vi "SMO.BasicByRef.GetValue.vi"(8 "error in (no error)":errorcluster, 11 "SMO.BasicByRef":refnum<class "SMO.BasicByRef.lvclass">) -> (0 "error out":errorcluster, 2 "Value":T1, 3 "SMO.BasicByRef out":refnum<class "SMO.BasicByRef.lvclass">)   [LabVIEW 2019, in "SMO.BasicByRef.lvclass"]
doc: "---------------------------------------------------------------\nJKI State Machine Objects™\nhttp://jki.net/state-machine-objects/\nCopyright (C) 2005-2015, JKI <info@jki.net>\nALL RIGHTS RESERVEDJKI State Machine Objects (SMO) 1.0.0.5\nJKI - JKI\nCopyright (c) 2016, JKI"
uses:
  SMO.BasicByRef.lvclass
  Typedefs/Value.ctl
  SMO.BasicByRef.lvclass/SMO.BasicByRef.ctl
panel:
  # "For instructions on how to use the JKI State Machine Objects, examples and video tutorials, visit:\nhttp://jki.net/state-machine-objects/\n\nJKI State Machine Objects™\nhttp://jki.net/state-machine-objects/\nCopyright (C) 2005-2015, JKI <info@jki.net>\nALL RIGHTS RESERVED"
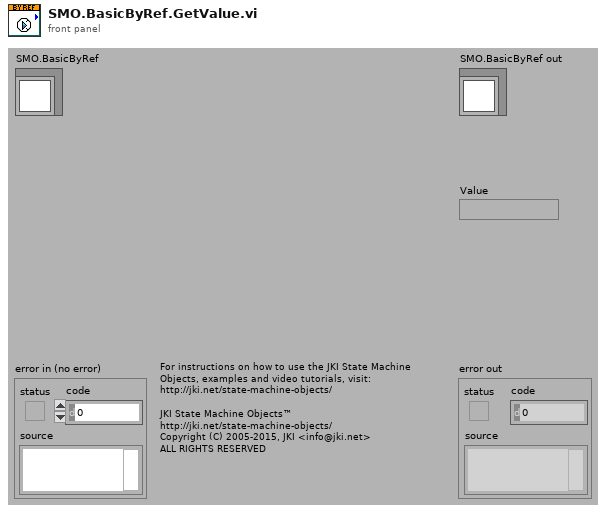
[diagram p1: front panel]
types:
  T1 = typedef "SMO.BasicByRef.lvclass/Value.ctl" = string
  T2 = typedef "SMO.BasicByRef.lvclass/PrivateData--Ref.ctl" = refnum<data-value>
  T3 = typedef "SMO.BasicByRef.lvclass/PrivateData--Cluster.ctl" = cluster{"Public Events":T4, "Protected Events":T5, "Private Events":T6, "Value":T1}
  T4 = typedef "SMO.BasicByRef.lvclass/PublicEvents--Cluster.ctl" = cluster{"Value Changed":refnum<user-event>}
  T5 = typedef "SMO.BasicByRef.lvclass/ProtectedEvents--Cluster.ctl" = cluster{"placeholder":refnum<user-event>}
  T6 = typedef "SMO.BasicByRef.lvclass/PrivateEvents--Cluster.ctl" = cluster{"New Value":refnum<user-event>}
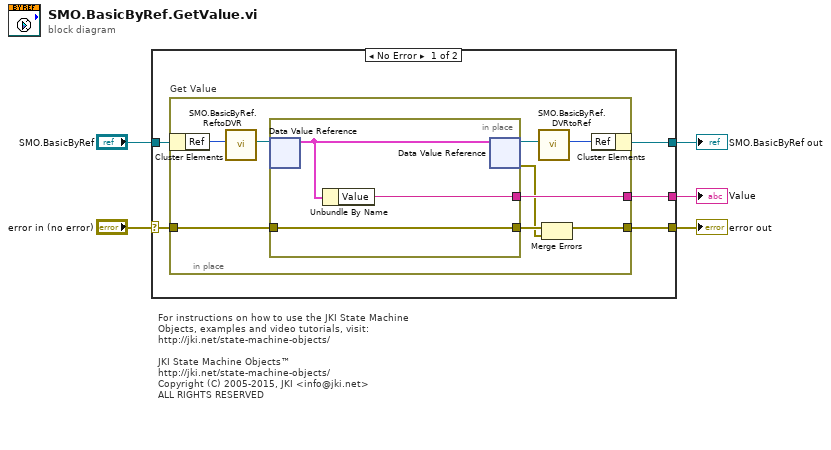
[diagram p0: block diagram]
diagram:
  # "For instructions on how to use the JKI State Machine Objects, examples and video tutorials, visit:\nhttp://jki.net/state-machine-objects/\n\nJKI State Machine Objects™\nhttp://jki.net/state-machine-objects/\nCopyright (C) 2005-2015, JKI <info@jki.net>\nALL RIGHTS RESERVED"
  n1 = case shown="No Error" "error in (no error)" {
    selector: "error in (no error)" -> [w8 w23]
    tunnel: "SMO.BasicByRef" -> [w9 w24]
    tunnel: [w6 w23] -> w4
    tunnel: [w7 w24] -> w3
    tunnel: [w10 _] -> w1
    frame No Error {
      n2 = in-place "Get Value" {
        in-place-border: w8 -> [w19]
        in-place-border: [w17] -> w6
        in-place-border: [w16] -> w10
        n3 = in-place-cluster #1(w9) -> ("Ref"=w15:u32)
        n4 = call "SMO.BasicByRef.ReftoDVR.vi"("Ref"=w15) -> ("Ref"=w14:T2)  [unwired: 10 in]
        n5 = in-place {
          in-place-border: w19 -> [w22]
          in-place-border: [w22] -> w18
          in-place-border: [w20] -> w16
          n6 = in-place-dvr #2(w14) -> (w21:T3)  [unwired: 1 out]
          n7 = Unbundle By Name(w21) -> ("Value"=w20:T1)
          n8 = in-place-dvr #2(w21) -> (w13:T2, w11:errorcluster)
        }
        n9 = call "SMO.BasicByRef.DVRtoRef.vi"("Ref"=w13) -> ("Ref"=w12:u32)  [unwired: 10 in]
        n10 = Merge Errors(w18, w11) -> (w17:errorcluster)
        n11 = in-place-cluster #1("Ref"=w12) -> (w7:refnum<class "SMO.BasicByRef.lvclass">)
      }
    }
    frame Error {
    }
  }
  "error out" <- w4
  "SMO.BasicByRef out" <- w3
  "Value" <- w1
